vi "TIO Device Init_Ser.vi"(8 "error in (no error)":errorcluster, 9 "ID":string="Twinleaf", 11 "Nom de ressource VISA":refnum<visa-resource-name>) -> (0 "error out":errorcluster={"status"=TRUE, "code"=-1073807252, "source"="VISA Read in SLIP Decode Serial Read.vi->NN VISA Read.vi->NN RPC.vi"}, 2 "ID Verified":bool, 3 "Nom de ressource VISA Out":refnum<visa-resource-name>, 4 "ID Verified":string)   [LabVIEW 2010]
uses:
  <vilib>/Instr/_visa.llb/VISA Configure Serial Port (Instr).vi
panel:
  # "TIO Init"
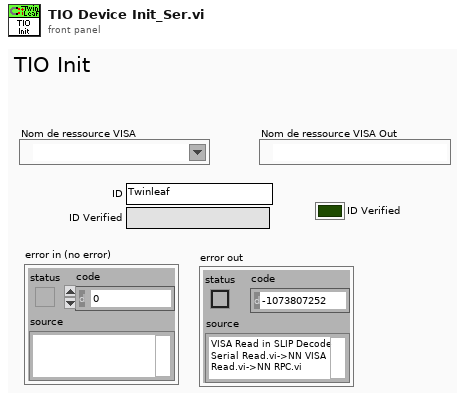
[diagram p1: front panel]
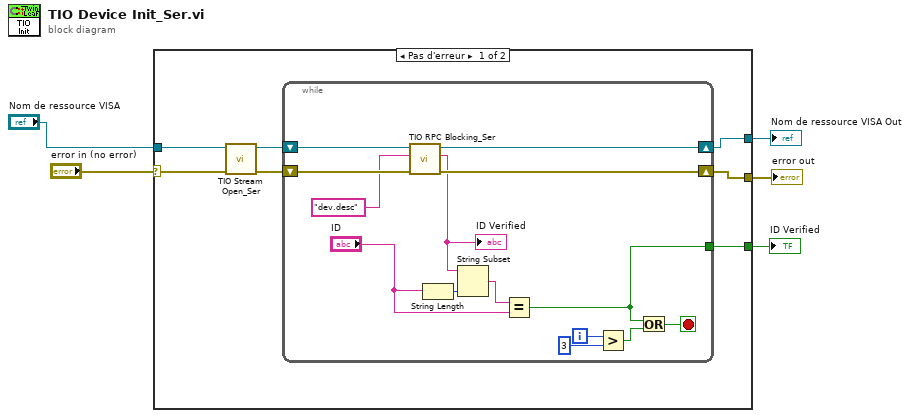
[diagram p0: block diagram]
diagram:
  n1 = case shown="Pas d'erreur" "error in (no error)" {
    selector: "error in (no error)" -> [w7 w28]
    tunnel: [w10 w27] -> w5
    tunnel: [w9 w28] -> w4
    tunnel: [w8 _] -> w3
    tunnel: "Nom de ressource VISA" -> [w6 w27]
    frame No Error {
      n2 = call <userlib>:"TIO Stream Open_Ser.vi"("error in (no error)"=w7, "Nom de ressource VISA"=w6) -> ("error out"=w11:errorcluster, "Nom de ressource VISA Out"=w12:refnum<visa-resource-name>)  [unwired: 7 in, 1 out]
      n3 = while {
        shift-right: [w25] -> w10
        shift-left: w12 -> [w14]
        shift-right: [w26] -> w9
        shift-left: w11 -> [w24]
        tunnel: [w13] -> w8
        i -> [w18]
        stop <- w15 stop-if-true
        n4 = call <userlib>:"TIO RPC Blocking_Ser.vi"("error in (no error)"=w24, "Named Method"="dev.desc" ("Topic"), "Nom de ressource VISA"=w14) -> ("error out"=w26:errorcluster, "Respose"=w21:string, "Nom de ressource VISA Out"=w25:refnum<visa-resource-name>)  [unwired: 5 in, 1 out]
        "ID Verified" <- w21
        n5 = String Length(string="ID") -> (length=w22:i32)
        n6 = String Subset(string=w21, length (rest)=w22) -> (substring=w20:string)  [unwired: 1 in]
        n7 = Equal?(x=w20, y="ID") -> (x = y?=w13:bool)
        n8 = Greater?(x=w18, y=3) -> (0:w16:bool)
        n9 = Or(x=w13, y=w16) -> (x .or. y?=w15:bool)
      }
    }
    frame Error {
    }
  }
  "error out" <- w4
  "Nom de ressource VISA Out" <- w5
  "ID Verified" <- w3
